vi "Build Elf Claim Matrix.vi"(8 "Error In":errorcluster, 11 "Elf Claim":string) -> (0 "Error Out":errorcluster, 1 "Elf Claim Matrix":T1, 2 "Distance from Top Edge":i32, 3 "Distance from Left Edge":i32, 4 "Width of Claim":i32, 5 "Height of Claim":i32)   [LabVIEW 2019]
doc: "Given a delimited elf claim (e.g. 1,2,3,4), build the claim matrix that will be added back onto the main fabric matrix. \n\nUsing the example (1,2,3,4), this would build a 3x4 matrix initialized with 1s."
uses:
  <vilib>/silver_ctls/ArrayMatrixCluster/Real Matrix NI_Silver.ctl
  <vilib>/Analysis/Matrix/Datatypes/RealMatrix.ctl
  <vilib>/Analysis/Matrix/Numeric/Add/Add (Elementwise) - RM,R.vi
  <vilib>/Analysis/Matrix/NI_Matrix.lvlib
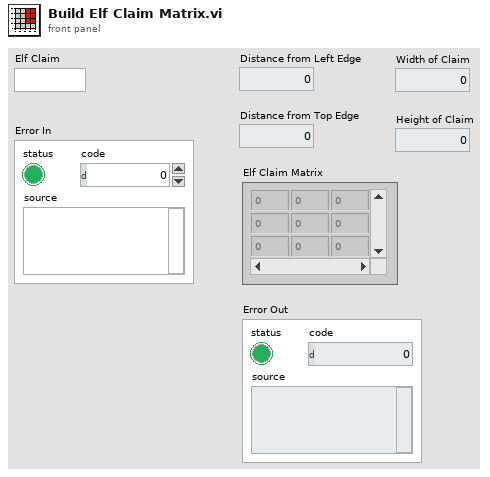
[diagram p1: front panel]
types:
  T1 = typedef "Real Matrix NI_Silver.ctl" = dbl[][]
  T2 = typedef "NI_Matrix.lvlib/RealMatrix.ctl" = dbl[][]
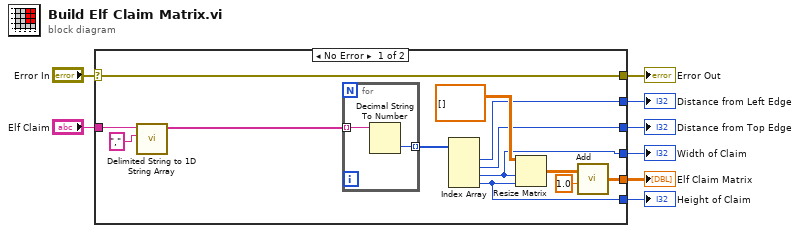
[diagram p0: block diagram]
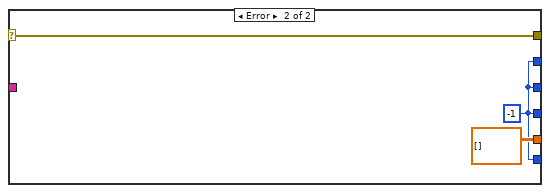
[diagram p2: hidden frame]
diagram:
  n1 = case shown="No Error" "Error In" {
    selector: "Error In" -> [w14 w26]
    tunnel: [w21 T2 [] ("A + c")] -> w4
    tunnel: [w17 w24] -> w8
    tunnel: [w16 w24] -> w7
    tunnel: "Elf Claim" -> [w13 _]
    tunnel: [w14 w26] -> w5
    tunnel: [w10 w24] -> w2
    tunnel: [w9 w24] -> w1
    frame No Error {
      n2 = call <vilib>:"Delimited String to 1D String Array.vi"("delimiter"=",", "delimited string"=w13) -> ("string array"=w11:string[])  [unwired: 9 in]
      n3 = for {
        tunnel: w11 -> [w23] mode=indexing
        tunnel: [w22] -> w15 mode=indexing
        n4 = Decimal String To Number(string=w23) -> (number=w22:i32)  [unwired: 2 in, 1 out]
      }
      n5 = Index Array(array=w15) -> (element #1=w16:i32, element #2=w17:i32, element #3=w10:i32, element #4=w9:i32)  [unwired: 4 in]
      n6 = Resize Matrix(1:w9, 2:w10, 4:T2 [] ("matrix")) -> (0:w19:T2)
      n7 = call-poly <vilib>:"Add.vi"("Real Scalar c"=1.0, "Real Matrix A"=w19) -> ("A + c"=w21:T2)
    }
    frame Error {
      w24 = -1
    }
  }
  "Distance from Top Edge" <- w8
  "Distance from Left Edge" <- w7
  "Elf Claim Matrix" <- w4
  "Error Out" <- w5
  "Width of Claim" <- w2
  "Height of Claim" <- w1
